vi "CAL-Plot Data.vi"(0 "Path":path, 1 "Mag graph":refnum<vi>, 5 "Name":string, 9 "Plot.Line Width":u8=2, 11 "error in (no error)":errorcluster) -> (4 "Path (out)":path, 15 "error out":errorcluster)   [LabVIEW 2020]
doc: "This helper VI loads calibration data from a file, and plots the magnitude and phase on graphs whose references are inputs to the VI. Handles the logic of overplotting data, selecting the colors and linestyles, and inserting the filename into the legend.\n\nKEH 9/10/09"
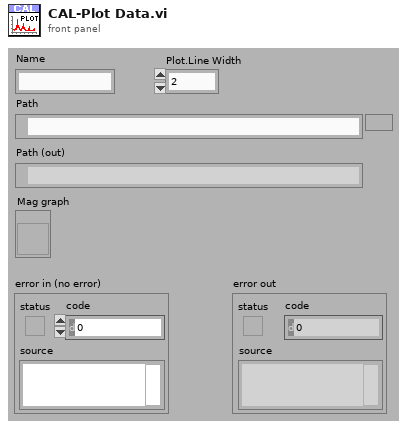
[diagram p1: front panel]
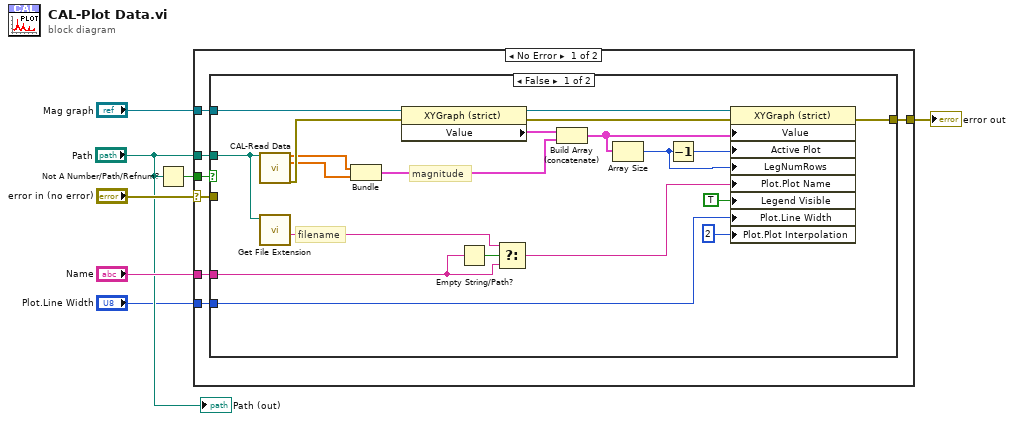
[diagram p0: block diagram]
diagram:
  n1 = Not A Number/Path/Refnum?(number/path/refnum="Path") -> (NaN/Path/Refnum?=w5:bool)
  n2 = case shown="No Error" "error in (no error)" {
    selector: "error in (no error)" -> [w11 w36]
    tunnel: "Mag graph" -> [w14 _]
    tunnel: [w13 w36] -> w6
    tunnel: w5 -> [w12 _]
    tunnel: "Path" -> [w8 _]
    tunnel: "Name" -> [w10 _]
    tunnel: "Plot.Line Width" -> [w9 _]
    frame No Error {
      n3 = case shown="False" w12 {
        tunnel: w14 -> [w34 _]
        tunnel: w11 -> [_ w35]
        tunnel: [w15 w35] -> w13
        tunnel: w10 -> [w18 _]
        tunnel: w8 -> [w17 _]
        tunnel: w9 -> [w16 _]
        frame False {
          # "filename"
          # "magnitude"
          n4 = call "CAL-Read Data.vi"("user path"=w17) -> ("Frequency (Hz)"=w30:dbl[], "Mag"=w29:dbl[], "error out"=w33:errorcluster)  [unwired: 10 in, 2 out]
          n5 = call <vilib>:"Get File Extension.vi"("file"=w17) -> ("filename without extension"=w19:string)  [unwired: 6 in, 4 out]
          n6 = Bundle("Frequency (Hz)"=w30, "Mag"=w29) -> (w31:cluster{"Frequency (Hz)":dbl[], "Mag":dbl[]})  [unwired: 1 in]
          n7 = property class="XYGraph (strict)"(reference=w34, error in=w33) -> (reference out=w27:refnum<vi>, error out=w26:errorcluster, "Value"=w32:cluster{"PTC Mag":dbl[], "PTC Phase":dbl[]}[])
          n8 = Empty String/Path?(string/path=w18) -> (empty?=w28:bool)
          n9 = Select(t=w19, s=w28, f=w18) -> (s? t:f=w22:string)
          n10 = Build Array (concatenate)(w32, w31) -> (w25:cluster{"Frequency (Hz)":dbl[], "Mag":dbl[]}[])
          n11 = Array Size(array=w25) -> (size(s)=w23:i32)
          n12 = Decrement(x=w23) -> (x-1=w24:i32)
          n13 = property class="XYGraph (strict)"(reference=w27, error in=w26, "Value"=w25, "Active Plot"=w24, "LegNumRows"=w23, "Plot.Plot Name"=w22, "Legend Visible"=TRUE ("Legend:Visible"), "Plot.Line Width"=w16, "Plot.Plot Interpolation"=u8 2) -> (error out=w15:errorcluster)  [unwired: 1 out]
        }
        frame True {
        }
      }
    }
    frame Error {
    }
  }
  "error out" <- w6
  "Path (out)" <- "Path"
